vi "RunTimeMenu Change GUID_Enable.vi"(8 "error in (no error)":errorcluster, 11 "Node Ptr":u64 format="%.0x") -> (0 "error out":errorcluster)   [LabVIEW 2010, in "Sensor Simulation Custom Device.lvlib"]
uses:
  Sensor Simulation Custom Device.lvlib
  Global.vi
  <vilib>/NI Veristand/Custom Device API/Custom Device API.lvlib
panel:
  in  "Tag":string
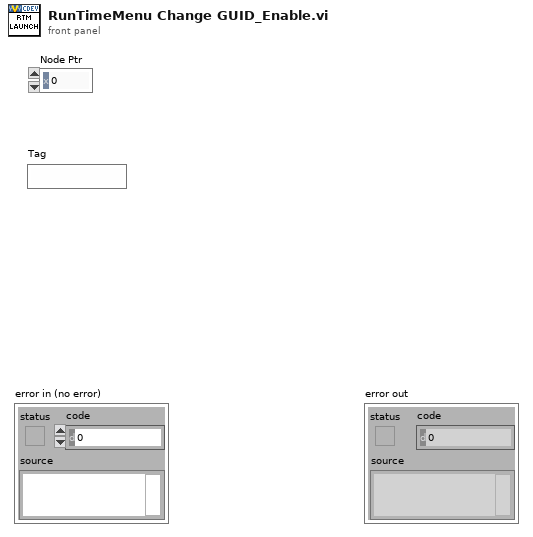
[diagram p1: front panel]
types:
  T1 = typedef "Custom Device API.lvlib/Custom Device Item Ref.ctl" = u64
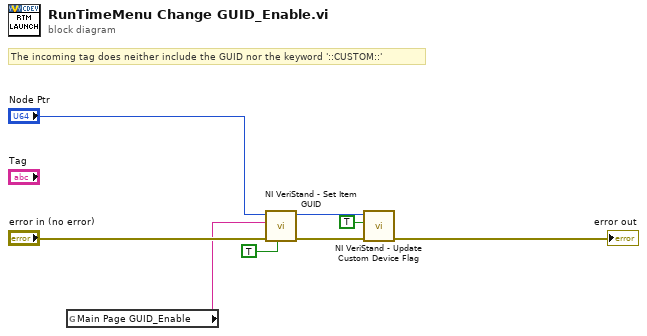
[diagram p0: block diagram]
diagram:
  # "The incoming tag does neither include the GUID nor the keyword '::CUSTOM::'"
  n1 = global read "Global.vi" "Main Page GUID_Enable"() -> (w1:string)
  n2 = call <vilib>:"NI VeriStand - Set Item GUID.vi"("Refresh System Explorer Tree? (F)"=TRUE, "error in (no error)"="error in (no error)", "GUID"=w1, "Item Ref in"="Node Ptr") -> ("error out"=w6:errorcluster, "Item Ref out"=w5:T1)  [unwired: 6 in]
  n3 = call <vilib>:"NI VeriStand - Update Custom Device Flag.vi"("error in (no error)"=w6, "Is Custom Device Active?"=TRUE, "Item Ref in"=w5) -> ("error out"=→"error out":errorcluster)  [unwired: 7 in, 1 out]
